vi "Multi-Point Tracking.vi"() -> ()   [LabVIEW 2021]
uses:
  <vilib>/myRIO/Instrument Drivers/Onboard IO/I2C/typedefs/I2C User Configuration.ctl
  <vilib>/myRIO/Instrument Drivers/Onboard IO/I2C/typedefs/I2C Transfer Rate.ctl
  <vilib>/myRIO/Instrument Drivers/Onboard IO/I2C/typedefs/I2C Reference.ctl
  <vilib>/myRIO/Common/Instrument Driver Framework/Utilities/typedefs/myRIO Generic Hardware Reference.ctl
  <vilib>/myRIO/Common/Instrument Driver Framework/Utilities/typedefs/Hardware Version Enum.ctl
  <vilib>/myRIO/Common/Instrument Driver Framework/Utilities/typedefs/myRIO v1.0 Reference.ctl
  <vilib>/myRIO/Common/Instrument Driver Framework/Utilities/typedefs/Generic FPGA Reference.ctl
  <vilib>/myRIO/Common/Instrument Driver Framework/myRIO v1.0/I2C/typedefs/I2C Channels Enum.ctl
  <vilib>/myRIO/Instrument Drivers/Onboard IO/I2C/typedefs/I2C Configuration.ctl
  <vilib>/userDefined/High Color/nirio_resource_hc.ctl
  <vilib>/myRIO/Instrument Drivers/Onboard IO/PWM/typedefs/PWM Reference.ctl
  <vilib>/myRIO/Common/Instrument Driver Framework/myRIO v1.0/PWM/typedefs/PWM Channels Enum.ctl
  <vilib>/myRIO/Instrument Drivers/Onboard IO/PWM/typedefs/PWM Configuration.ctl
  <vilib>/myRIO/Common/Instrument Driver Framework/myRIO v1.0/Encoder/typedefs/Encoder Signal Mode.ctl
  <vilib>/myRIO/Instrument Drivers/Onboard IO/Encoder/typedefs/Encoder Reference.ctl
  <vilib>/myRIO/Common/Instrument Driver Framework/myRIO v1.0/Encoder/typedefs/Encoder Channels Enum.ctl
  <vilib>/myRIO/Common/Instrument Driver Framework/myRIO v1.0/Encoder/typedefs/Encoder Configuration v1.0.ctl
  <vilib>/myRIO/Instrument Drivers/Onboard IO/DIO/typedefs/DIO Reference.ctl
  <vilib>/myRIO/Common/Instrument Driver Framework/myRIO v1.0/DIO/typedefs/DIO Channels List.ctl
  <vilib>/myRIO/Common/Instrument Driver Framework/myRIO v1.0/DIO/typedefs/DIO Channels Enum.ctl
  <vilib>/myRIO/Common/Instrument Driver Framework/Utilities/vis/Is FPGA Ref Available.vi
  <vilib>/myRIO/Common/Instrument Driver Framework/myRIO v1.0/I2C/vis/myRIO v1.1 Open I2C.vi
  <vilib>/myRIO/Instrument Drivers/Onboard IO/I2C/vis/Configure.vi
  <vilib>/myRIO/Instrument Drivers/Onboard IO/I2C/vis/Write.vi
  <vilib>/myRIO/Common/Instrument Driver Framework/myRIO v1.0/Encoder/vis/myRIO v1.1 Open Encoder.vi
  <vilib>/myRIO/Instrument Drivers/Onboard IO/Encoder/vis/Read.vi
  <vilib>/myRIO/Common/Instrument Driver Framework/myRIO v1.0/PWM/vis/myRIO v1.1 Open PWM.vi
  <vilib>/myRIO/Instrument Drivers/Onboard IO/PWM/vis/Set Duty Cycle and Frequency.vi
  <vilib>/myRIO/Common/Instrument Driver Framework/myRIO v1.0/DIO/vis/myRIO v1.1 Open DIO.vi
  <vilib>/myRIO/Instrument Drivers/Onboard IO/DIO/vis/Write.vi
  <vilib>/myRIO/Instrument Drivers/Onboard IO/I2C/vis/Write Read.vi
  <vilib>/Analysis/baseanly.llb/Mean (DBL).vi
  <vilib>/myRIO/Common/Instrument Driver Framework/Utilities/vis/Validate Channels.vi
  <vilib>/myRIO/Common/Instrument Driver Framework/myRIO v1.0/I2C/vis/myRIO v1.0 Reserve I2C.vi
  <vilib>/myRIO/Common/Instrument Driver Framework/myRIO v1.0/Encoder/vis/myRIO v1.0 Reserve Encoder.vi
  <vilib>/myRIO/Common/Instrument Driver Framework/myRIO v1.0/PWM/vis/myRIO v1.0 Reserve PWM.vi
  <vilib>/myRIO/Common/Instrument Driver Framework/myRIO v1.0/DIO/vis/myRIO v1.0 Reserve DIO.vi
  <vilib>/myRIO/Common/Instrument Driver Framework/myRIO v1.0/UART/vis/myRIO v1.0 Close UART.vi
  <vilib>/myRIO/Common/Instrument Driver Framework/myRIO v1.0/I2C/vis/myRIO v1.0 Build MUX Configuration I2C.vi
  <vilib>/myRIO/Common/Instrument Driver Framework/myRIO v1.0/Resource Manager/vis/myRIO v1.0 Reserve Channel List.vi
  <vilib>/myRIO/Common/Instrument Driver Framework/myRIO v1.0/Encoder/vis/myRIO v1.0 Build MUX Configuration Encoder.vi
  <vilib>/myRIO/Common/Instrument Driver Framework/myRIO v1.0/PWM/vis/myRIO v1.0 Build MUX Configuration PWM.vi
  <vilib>/myRIO/Common/Instrument Driver Framework/myRIO v1.0/DIO/vis/myRIO v1.0 Build MUX Configuration DIO.vi
  <vilib>/myRIO/Common/Instrument Driver Framework/myRIO v1.0/Resource Manager/vis/myRIO v1.0 Create Configuration List.vi
  <vilib>/myRIO/Common/Instrument Driver Framework/myRIO v1.0/Resource Manager/vis/myRIO v1.0 Reserve Channel.vi
  <vilib>/myRIO/Common/Instrument Driver Framework/myRIO v1.0/Resource Manager/vis/myRIO v1.0 Unreserve Channel.vi
  <vilib>/myRIO/Common/Instrument Driver Framework/myRIO v1.0/Resource Manager/vis/myRIO v1.0 Build Mutex Name.vi
  <vilib>/Utility/VariantDataType/GetNumericInfo.vi
  <vilib>/Utility/error.llb/Error Cluster From Error Code.vi
  <vilib>/myRIO/Common/Instrument Driver Framework/myRIO v1.0/myRIO v1.1 Open.vi
  <vilib>/myRIO/Common/Instrument Driver Framework/Utilities/vis/IO Manager.vi
  <vilib>/myRIO/Common/Instrument Driver Framework/Utilities/vis/Configuration Manager.vi
  <vilib>/myRIO/Common/Instrument Driver Framework/myRIO v1.0/Resource Manager/vis/myRIO v1.0 Configure IO.vi
  <vilib>/myRIO/Common/Instrument Driver Framework/myRIO v1.0/myRIO v1.0 Close.vi
  <vilib>/myRIO/Common/Instrument Driver Framework/myRIO v1.0/I2C/vis/myRIO v1.0 Configure I2C.vi
  <vilib>/myRIO/Common/Instrument Driver Framework/myRIO v1.0/I2C/vis/myRIO v1.0 Write I2C.vi
  <vilib>/myRIO/Common/Instrument Driver Framework/myRIO v1.0/Encoder/vis/myRIO v1.0 Configure Encoder.vi
  <vilib>/myRIO/Common/Instrument Driver Framework/myRIO v1.0/Encoder/vis/myRIO v1.0 Read Encoder.vi
  <vilib>/addons/Fuzzy Logic/FL Fuzzy Controller (SISO).vi
  <vilib>/myRIO/Common/Instrument Driver Framework/myRIO v1.0/PWM/vis/myRIO v1.0 Write PWM.vi
  <vilib>/myRIO/Common/Instrument Driver Framework/myRIO v1.0/DIO/vis/myRIO v1.0 Write DIO.vi
  <vilib>/myRIO/Common/Instrument Driver Framework/myRIO v1.0/I2C/vis/myRIO v1.0 Read I2C.vi
  <vilib>/myRIO/Common/Instrument Driver Framework/Utilities/vis/FPGA Ref Manager.vi
  <vilib>/myRIO/Common/Instrument Driver Framework/myRIO v1.0/myRIO v1.0 Reset FPGA.vi
  <vilib>/myRIO/Common/Instrument Driver Framework/myRIO v1.0/IRQ/vis/myRIO v1.0 IRQ Info FGV.vi
  <vilib>/myRIO/Common/Instrument Driver Framework/myRIO v1.0/IRQ/vis/myRIO v1.0 Timer IRQ Info FGV.vi
  <vilib>/myRIO/Common/Instrument Driver Framework/myRIO v1.0/IRQ/vis/myRIO v1.0 ISR Agent.vi
  <vilib>/myRIO/Instrument Drivers/Utilities/vis/Reset Index.vi
  <vilib>/myRIO/Common/Instrument Driver Framework/myRIO v1.0/Resource Manager/vis/myRIO v1.0 Block Write Resource Manager.vi
  <vilib>/myRIO/Express VI/Onboard IO/I2C/I2C Express VI.xnode
  <vilib>/myRIO/Instrument Drivers/Onboard IO/I2C/vis/myRIO I2C Open.xnode
  <vilib>/myRIO/Express VI/Onboard IO/Encoder/Encoder Express VI.xnode
  <vilib>/myRIO/Instrument Drivers/Onboard IO/Encoder/vis/myRIO Encoder Open.xnode
  <vilib>/myRIO/Common/Instrument Driver Framework/myRIO v1.0/Encoder/typedefs/Encoder Count Direction Enum.ctl
  <vilib>/myRIO/Express VI/Onboard IO/PWM/PWM Express VI.xnode
  <vilib>/myRIO/Instrument Drivers/Onboard IO/PWM/vis/myRIO PWM Open.xnode
  <vilib>/myRIO/Express VI/Onboard IO/DO/DO Express VI.xnode
  <vilib>/myRIO/Instrument Drivers/Onboard IO/DIO/vis/myRIO DIO Open.xnode
  <vilib>/myRIO/Instrument Drivers/Onboard IO/I2C/I2C.lvlib
  <vilib>/ptbypt/NI_PtbyPt.lvlib
  <vilib>/myRIO/Instrument Drivers/Onboard IO/PWM/PWM.lvlib
  <vilib>/myRIO/Instrument Drivers/Onboard IO/DIO/DIO.lvlib
  <vilib>/myRIO/Instrument Drivers/Utilities/Utilities.lvlib
  <vilib>/myRIO/Instrument Drivers/Onboard IO/Encoder/Encoder.lvlib
  <vilib>/Analysis/NI_AALBase.lvlib
  <vilib>/addons/Fuzzy Logic/NI_Fuzzy_Logic_API.lvlib
panel:
  out "correct gz":dbl
  out "correct GZ":dbl format="%0.2f"
  out "速度":dbl
  out "單位距離":dbl
  out "總行程":dbl
  out "右圈數":dbl
  out "左圈數":dbl
  out "Reset counter":bool
  out "Velocity(cm/sec)":cluster{dbl[], dbl[]}(graph)
  in  "array":dbl[][](array[numeric])
  out "output cluster":cluster{"Array 2":dbl[], "Array 2":dbl[]}
  out "appended array":dbl[][](array[numeric])
  out "path5":cluster{dbl[], dbl[]}(graph)
  out "distance":dbl
  out "Yaw target":dbl
  out "Yt":dbl
  out "Xt":dbl
  out "Yg":dbl
  out "Xg":dbl
  out "P-gain":dbl
  out "Error":cluster{dbl[], dbl[]}(graph)
  out "Yaw error":dbl
  out "Command/Gauge":cluster{dbl[], dbl[]}[](graph)
  out "angular degree":dbl format="%0.2f"
  out "Velocity duty cycle":dbl(slide) scale=0.0..1.0
  out "Turn duty cycle":dbl(slide) scale=0.0..1.0
  in  "start":bool
  in  "remote":bool
  out "Guage":dbl(knob) scale=0.0..360.0
  out "GZ":dbl format="%0.2f"
  in  "G 歸零":bool
  in  "G 校正":bool
  in  "stop":bool
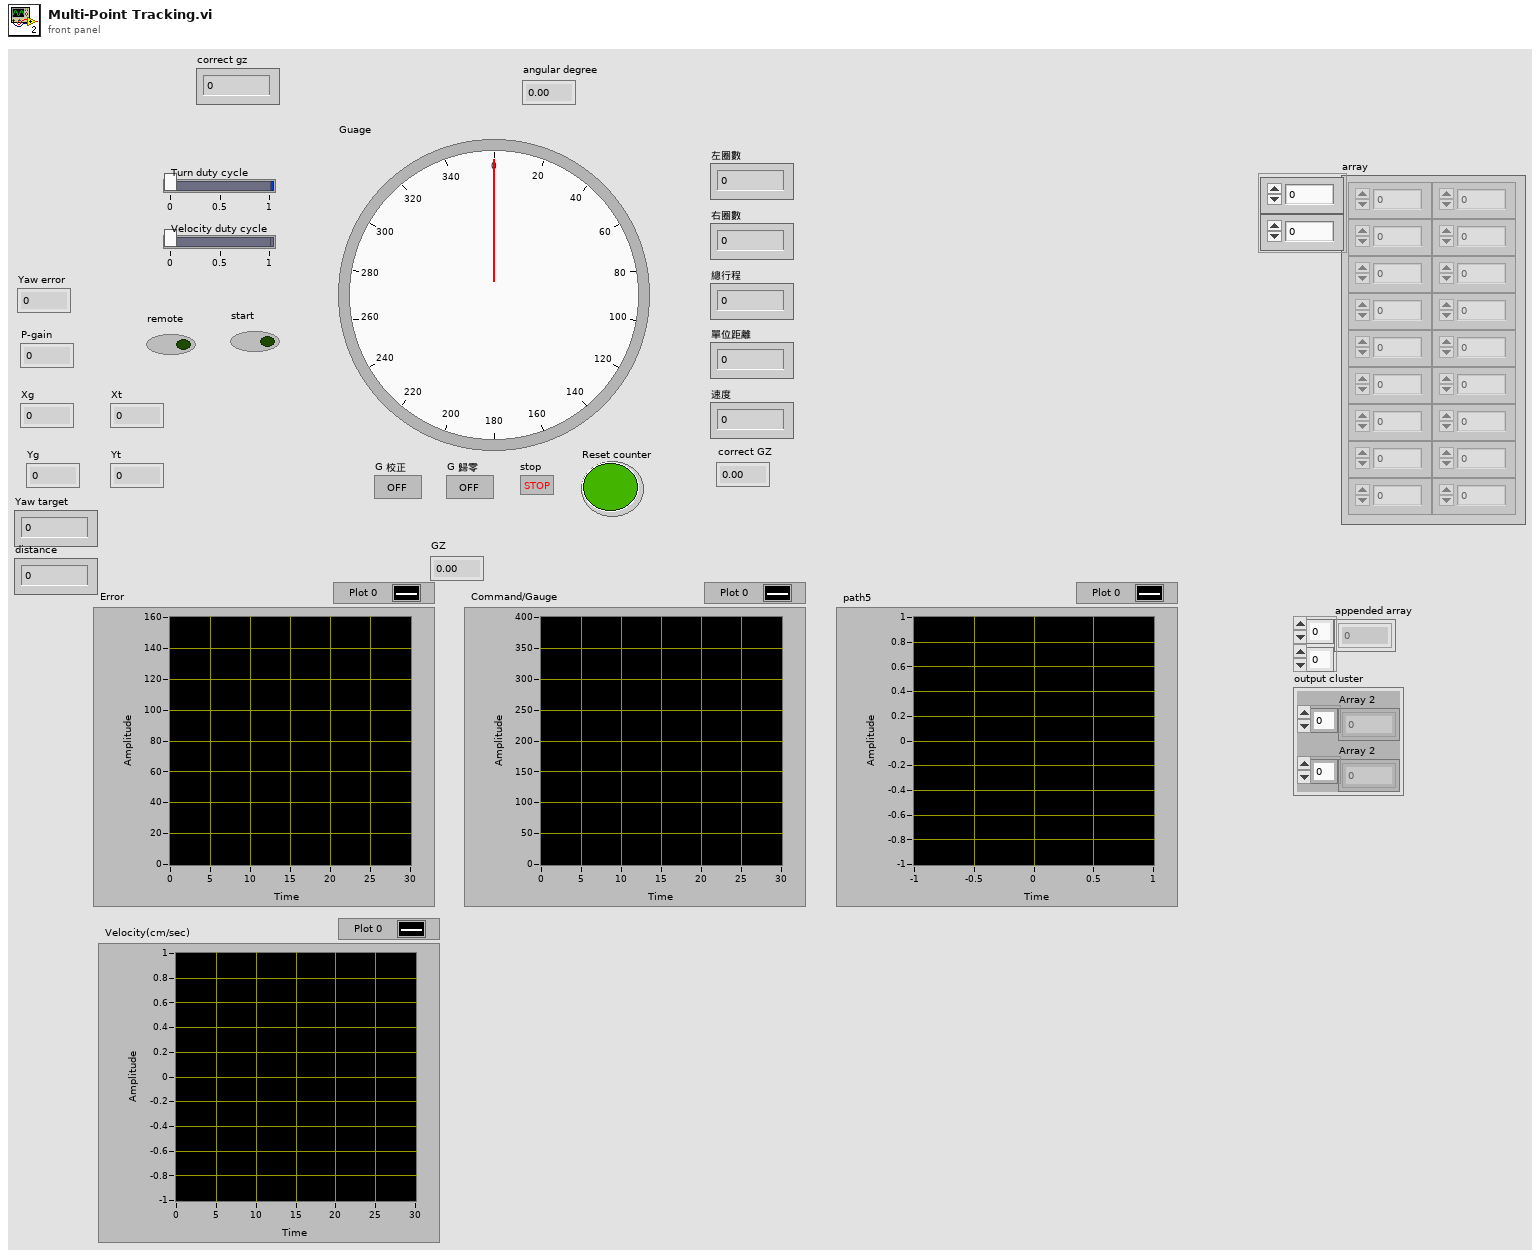
[diagram p1: front panel]
types:
  T1 = typedef "I2C.lvlib/I2C Reference.ctl" = cluster{"myRIO Reference":T2, "I2C Channels Enum":T6, "I2C Configuration":T7}
  T2 = typedef "myRIO Generic Hardware Reference.ctl" = cluster{"myRIO Model":T3, "myRIO Hardware Reference":T4}
  T3 = typedef "Hardware Version Enum.ctl" = enum16{"Unknown", "myRIO-1900", "myRIO-1950", "roboRIO", "NI ELVIS RIO CM", "ELVIS III"}
  T4 = typedef "myRIO v1.0 Reference.ctl" = cluster{"Generic FPGA Reference":T5, "Allow multiple opens":bool}
  T5 = typedef "Generic FPGA Reference.ctl" = refnum<k20>
  T6 = typedef "I2C Channels Enum.ctl" = enum16{"Not Connected", "A/I2C", "B/I2C", "I2C/I2C"}
  T7 = typedef "I2C.lvlib/I2C Configuration.ctl" = cluster{"I2C Transfer Rate":T8}
  T8 = typedef "I2C.lvlib/I2C Transfer Rate.ctl" = enum16{"Standard mode (100 kbps)", "Fast mode (400 kbps)"}
  T9 = typedef "I2C.lvlib/I2C User Configuration.ctl" = cluster{"I2C Transfer Rate":T8}
  T10 = typedef "nirio_resource_hc.ctl" = tag
  T11 = typedef "Encoder.lvlib/Encoder Reference.ctl" = cluster{"myRIO Reference":T2, "Encoder Channels Enum":T12}
  T12 = typedef "Encoder Channels Enum.ctl" = enum16{"Not Connected", "C/ENC0", "C/ENC1", "A/ENC", "A/ENC0", "A/ENC1", "A/ENC2", "A/ENC3", "A/ENC4", "A/ENC5", "A/ENC6", "A/ENC7", "A/ENC8", "A/ENC9", "B/ENC", "B/ENC0", "B/ENC1", "B/ENC2", "B/ENC3", "B/ENC4", "B/ENC5", "B/ENC6", "B/ENC7", "B/ENC8", "B/ENC9", "DIO/ENC0", "DIO/ENC1", "DIO/ENC2", "DIO/ENC3", "DIO/ENC4"}
  T13 = typedef "Encoder Signal Mode.ctl" = enum16{"Quadrature phase signal", "Step and direction signal"}
  T14 = typedef "DIO.lvlib/DIO Reference.ctl" = cluster{"myRIO Reference":T2, "DIO Channels List":T15}
  T15 = typedef "DIO Channels List.ctl" = T16[]
  T16 = typedef "DIO Channels Enum.ctl" = enum16{"Not Connected", "C/DIO0", "C/DIO1", "C/DIO2", "C/DIO3", "C/DIO4", "C/DIO5", "C/DIO6", "C/DIO7", "A/DIO0", "A/DIO1", "A/DIO2", "A/DIO3", "A/DIO4", "A/DIO5", "A/DIO6", "A/DIO7", "A/DIO8", "A/DIO9", "A/DIO10", "A/DIO11", "A/DIO12", "A/DIO13", "A/DIO14", "A/DIO15", "A/DIO16", "A/DIO17", "A/DIO18", "A/DIO19", "B/DIO0", "B/DIO1", "B/DIO2", "B/DIO3", "B/DIO4", "B/DIO5", "B/DIO6", "B/DIO7", "B/DIO8", "B/DIO9", "B/DIO10", "B/DIO11", "B/DIO12", "B/DIO13", "B/DIO14", "B/DIO15", "B/DIO16", "B/DIO17", "B/DIO18", "B/DIO19", "LED0", "LED1", "LED2", "LED3", "Button0", "DIO/DIO0", "DIO/DIO1", "DIO/DIO2", "DIO/DIO3", "DIO/DIO4", "DIO/DIO5", "DIO/DIO6", "DIO/DIO7", "DIO/DIO8", "DIO/DIO9", "SPI/CS0", "SPI/CS1", "SPI/CS2", "SPI/CS3", "LED RADIO (Green)", "LED RADIO (Red)", "LED COMM (Green)", "LED COMM (Red)", "LED MODE (Green)", "LED MODE (Red)"}
  T17 = typedef "PWM.lvlib/PWM Reference.ctl" = cluster{"myRIO Reference":T2, "PWM Channels Enum":T18, "PWM Configuration":T19}
  T18 = typedef "PWM Channels Enum.ctl" = enum16{"Not Connected", "C/PWM0", "C/PWM1", "A/PWM0", "A/PWM1", "A/PWM2", "A/PWM3", "A/PWM4", "A/PWM5", "A/PWM6", "A/PWM7", "A/PWM8", "A/PWM9", "A/PWM10", "A/PWM11", "A/PWM12", "A/PWM13", "A/PWM14", "A/PWM15", "A/PWM16", "A/PWM17", "A/PWM18", "A/PWM19", "B/PWM0", "B/PWM1", "B/PWM2", "B/PWM3", "B/PWM4", "B/PWM5", "B/PWM6", "B/PWM7", "B/PWM8", "B/PWM9", "B/PWM10", "B/PWM11", "B/PWM12", "B/PWM13", "B/PWM14", "B/PWM15", "B/PWM16", "B/PWM17", "B/PWM18", "B/PWM19", "PWM/PWM0", "PWM/PWM1", "PWM/PWM2", "PWM/PWM3", "PWM/PWM4", "PWM/PWM5", "PWM/PWM6", "PWM/PWM7", "PWM/PWM8", "PWM/PWM9"}
  T19 = typedef "PWM.lvlib/PWM Configuration.ctl" = cluster{"Frequency":dbl, "Duty Cycle":dbl}
  T20 = typedef "NI_Fuzzy_Logic_API.lvlib/FL System.ctl" = cluster{"input variables":T21[], "output variables":T21[], "rules":T24[], "defuzzification method":T30, "description":string, "user MF interpolating polynomials":T31[]}
  T21 = typedef "NI_Fuzzy_Logic_API.lvlib/FL Variable.ctl" = cluster{"name":string, "range":dbl[], "MFs":T22[]}
  T22 = typedef "NI_Fuzzy_Logic_API.lvlib/FL Membership Function.ctl" = cluster{"name":string, "shape":T23, "points":dbl[], "color":u32, "user-defined shape index":i32}
  T23 = typedef "NI_Fuzzy_Logic_API.lvlib/FL Membership Function Shape.ctl" = u16
  T24 = typedef "NI_Fuzzy_Logic_API.lvlib/FL Rule.ctl" = cluster{"antecedents":T25[], "antecedent connective":T27, "consequents":T28[], "consequent implication":T29, "degree of support":dbl}
  T25 = typedef "NI_Fuzzy_Logic_API.lvlib/FL Antecedent.ctl" = cluster{"Var Index":i32, "MF Index":i32, "Cond":T26}
  T26 = typedef "NI_Fuzzy_Logic_API.lvlib/FL Modifier.ctl" = u16
  T27 = typedef "NI_Fuzzy_Logic_API.lvlib/FL Antecedent Connective.ctl" = u16
  T28 = typedef "NI_Fuzzy_Logic_API.lvlib/FL Consequent.ctl" = cluster{"Var Index":i32, "MF Index":i32, "Cond":T26}
  T29 = typedef "NI_Fuzzy_Logic_API.lvlib/FL Consequent Implication.ctl" = u16
  T30 = typedef "NI_Fuzzy_Logic_API.lvlib/FL Defuzzification.ctl" = u16
  T31 = typedef "NI_Fuzzy_Logic_API.lvlib/FL Interpolating polynomials.ctl" = cluster{"X":dbl[], "Y":dbl[], "Y(x) coeff":dbl[][], "X(y) coeff":dbl[][], "Area(y) coeff":dbl[][], "coa_x(y) coeff":dbl[][]}
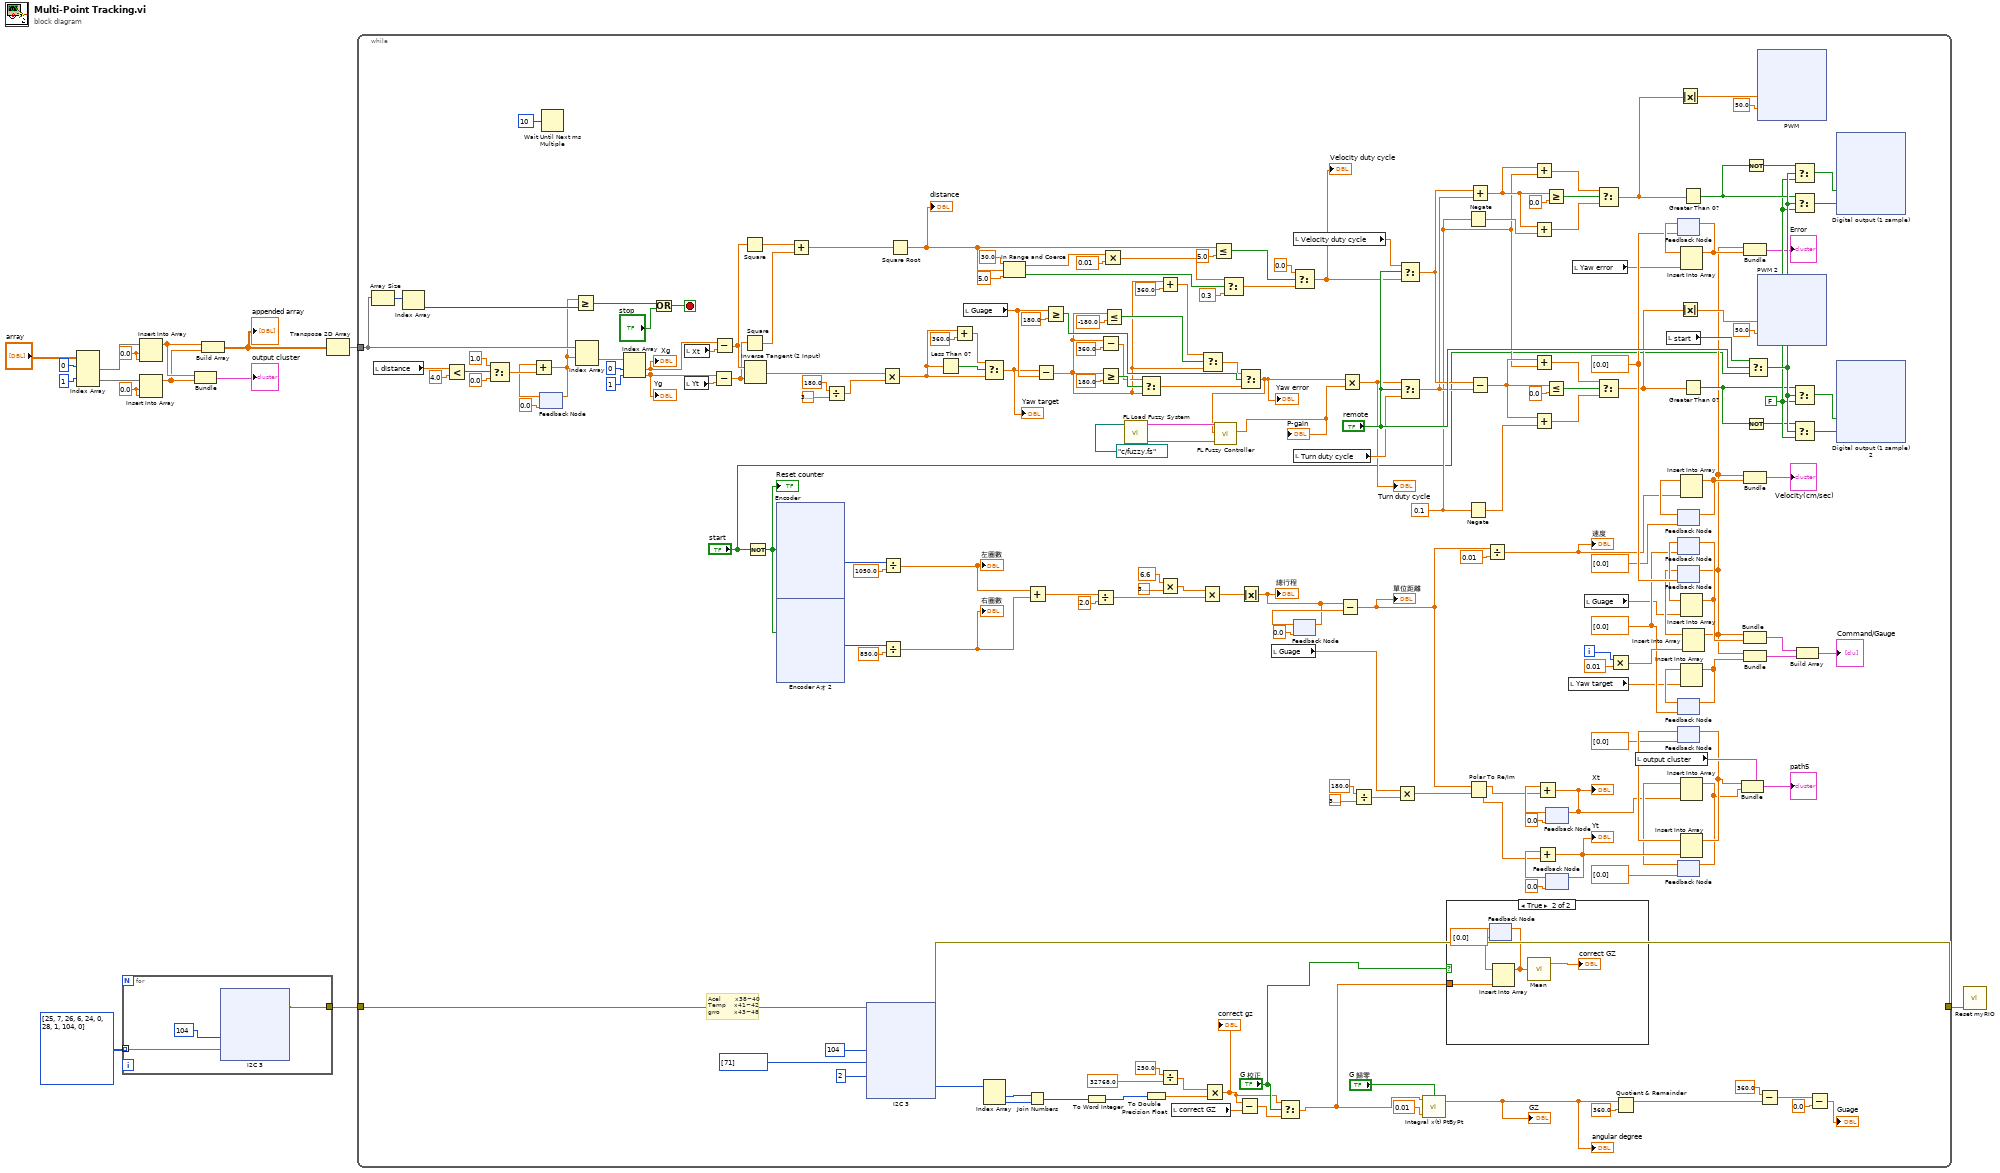
[diagram p0: block diagram]
diagram:
  w1 = 0.0 ("new element/subarray")
  w3 = 0.0 ("new element/subarray")
  n1 = Index Array(array="array", index (row) #1=0 ("index (row)"), index (row) #2=1 ("index (row)")) -> (element #1=w7:dbl[], element #2=w6:dbl[])  [unwired: 2 in]
  n2 = for {
    tunnel: u8[][] [[25, 7], [26, 6], [24, 0], [28, 1], [104, 0]] ("Bytes to Write") -> [w16] mode=indexing
    tunnel: [w18] -> w14
    n3 = xnode "I2C 3"("Slave Address (7-bit)"=u8 104, "Bytes to Write"=w16) -> ("error out"=w18:errorcluster)  [unwired: 1 in]
  }
  n4 = Insert Into Array(array=w7, index=w3, new element=w3) -> (w4:dbl[])
  n5 = Insert Into Array(array=w6, index=w1, new element=w1) -> (w2:dbl[])
  n6 = Bundle("array"=w4, "array"=w2) -> (→"output cluster":cluster{"array":dbl[], "array":dbl[]})  [unwired: 1 in]
  n7 = Build Array(w4, w2) -> (w12:dbl[][])
  "appended array" <- w12
  n8 = Transpose 2D Array(2D array=w12) -> (transposed array=w10:dbl[][])
  n9 = while {
    tunnel: w14 -> [w77]
    tunnel: [w76] -> w13
    tunnel: w10 -> [w117]
    i -> [w218]
    stop <- w242 stop-if-true
    w185 = 0.1 ("y")
    w220 = dbl[] [0.0]
    w225 = dbl[] [0.0]
    w232 = FALSE
    # "Acel       x38~40\nTemp    x41~42\ngrro       x43~48"
    n10 = Array Size(array=w117) -> (size(s)=w116:i32[])
    n11 = local read "distance"() -> (w127:dbl)
    n12 = Index Array(array=w116) -> (element=w115:i32)  [unwired: 1 in]
    n13 = Less?(x=w127, y=4.0) -> (x < y?=w125:bool)
    n14 = Select(t=1.0, s=w125, f=0.0) -> (s? t:f=w122:dbl)
    n15 = feedback #1(0.0) -> (w121:dbl)
    n16 = Add(x=w121, y=w122) -> (x+y=w114:dbl)
    n17 = feedback-in #1(w114) -> ()
    n18 = Wait Until Next ms Multiple(millisecond multiple=u32 10) -> ()  [unwired: 1 out]
    n19 = Greater Or Equal?(x=w114, y=w115) -> (x >= y?=w119:bool)
    n20 = Index Array(array=w117, index (row)=w114) -> (element=w118:dbl[])  [unwired: 1 in]
    n21 = Index Array(array=w118, index #1=0 ("index"), index #2=1 ("index")) -> (element #1=w111:dbl, element #2=w110:dbl)
    "Yg" <- w110
    "Xg" <- w111
    n22 = Or(x=w119, y="stop") -> (x .or. y?=w242:bool)
    n23 = local read "Xt"() -> (w171:dbl)
    n24 = local read "Yt"() -> (w170:dbl)
    n25 = Subtract(x=w110, y=w170) -> (x-y=w168:dbl)
    n26 = Subtract(x=w111, y=w171) -> (x-y=w169:dbl)
    n27 = Square(x=w169) -> (x^2=w167:dbl)
    n28 = Square(x=w168) -> (x^2=w166:dbl)
    n29 = Inverse Tangent (2 Input)(1:w168, 2:w169) -> (0:w164:dbl)
    n30 = Not(x="start") -> (.not. x?=w101:bool)
    "Reset counter" <- w101
    n31 = xnode "Encoder"("Reset Counter"=w101) -> ("Counter Value"=w97:i32)  [unwired: 1 in, 3 out]
    n32 = xnode "Encoder Aオ 2"("Reset Counter"=w101) -> ("Counter Value"=w98:i32)  [unwired: 1 in, 3 out]
    n33 = Add(x=w167, y=w166) -> (x+y=w165:dbl)
    n34 = Divide(x=180.0, y=3.141592653589793) -> (x/y=w161:dbl)
    n35 = xnode "I2C 3"("Slave Address (7-bit)"=u8 104, "Bytes to Write"=u8[] [71], "Byte Count"=u32 2, "error in (no error)"=w77) -> ("Bytes Read"=w72:u8[], "error out"=w76:errorcluster)
    n36 = Multiply(x=w164, y=w161) -> (x*y=w159:dbl)
    n37 = Divide(x=w97, y=1050.0) -> (x/y=w96:dbl)
    "左圈數" <- w96
    n38 = Divide(x=w98, y=850.0) -> (x/y=w95:dbl)
    "右圈數" <- w95
    n39 = Square Root(x=w165) -> (sqrt(x)=w148:dbl)
    "distance" <- w148
    n40 = Less Than 0?(x=w159) -> (x < 0?=w160:bool)
    n41 = Add(x=w159, y=360.0) -> (x+y=w157:dbl)
    n42 = local read "Guage"() -> (w172:dbl)
    n43 = Select(t=w157, s=w160, f=w159) -> (s? t:f=w156:dbl)
    "Yaw target" <- w156
    n44 = Index Array(array=w72) -> (element #1=w255:u8, element #2=w254:u8)  [unwired: 2 in]
    n45 = In Range and Coerce(upper limit=30.0, x=w148, lower limit=5.0) -> (coerced(x)=w153:dbl, In Range?=w151:bool)
    n46 = Add(x=w96, y=w95) -> (x+y=w94:dbl)
    n47 = Join Numbers(hi=w255, lo=w254) -> ((hi.lo)=w253:u16)
    n48 = Subtract(x=w156, y=w172) -> (x-y=w199:dbl)
    n49 = Greater Or Equal?(x=w172, y=180.0) -> (x >= y?=w205:bool)
    n50 = To Word Integer(number=w253) -> (16bit integer=w250:i16)
    n51 = Divide(x=w94, y=2.0) -> (x/y=w89:dbl)
    n52 = Subtract(x=w199, y=360.0) -> (x-y=w200:dbl)
    n53 = Greater Or Equal?(x=w199, y=180.0) -> (x >= y?=w207:bool)
    n54 = Multiply(x=w153, y=0.01) -> (x*y=w150:dbl)
    n55 = Less Or Equal?(x=w199, y=-180.0) -> (x <= y?=w208:bool)
    n56 = call <vilib>:"FL Load Fuzzy System.vi"("file path"=path "c:/fuzzy.fs") -> ("error out"=w64:errorcluster, "fuzzy system out"=w65:T20)  [unwired: 9 in]
    n57 = Select(t=w200, s=w207, f=w199) -> (s? t:f=w201:dbl)
    n58 = To Double Precision Float(number=w250) -> (double precision float=w243:dbl)
    n59 = Add(x=w199, y=360.0) -> (x+y=w198:dbl)
    n60 = Multiply(x=6.6, y=3.141592653589793) -> (x*y=w90:dbl)
    n61 = Divide(x=250.0, y=32768.0) -> (x/y=w249:dbl)
    n62 = local read "correct GZ"() -> (w70:dbl)
    n63 = Multiply(x=w90, y=w89) -> (x*y=w88:dbl)
    n64 = Select(t=w198, s=w208, f=w199) -> (s? t:f=w202:dbl)
    n65 = Multiply(x=w249, y=w243) -> (x*y=w68:dbl)
    "correct gz" <- w68
    n66 = Less Or Equal?(x=w148, y=5.0) -> (x <= y?=w146:bool)
    n67 = Select(t=w150, s=w151, f=0.3) -> (s? t:f=w145:dbl)
    n68 = Subtract(x=w68, y=w70) -> (x-y=w67:dbl)
    n69 = Select(t=w202, s=w205, f=w201) -> (s? t:f=w63:dbl)
    "Yaw error" <- w63
    n70 = call-poly <vilib>:"FL Fuzzy Controller.vi"("error in (no error)"=w64, "input value"=w63, "fuzzy system in"=w65) -> ("output value"=w62:dbl)  [unwired: 4 in, 4 out]
    "P-gain" <- w62
    n71 = Absolute Value(x=w88) -> (abs(x)=w85:dbl)
    "總行程" <- w85
    n72 = local read "Guage"() -> (w142:dbl)
    n73 = Select(t=w68, s="G 校正", f=w67) -> (s? t:f=w66:dbl)
    n74 = local read "Velocity duty cycle"() -> (w178:dbl)
    n75 = Select(t=0.0, s=w146, f=w145) -> (s? t:f=w143:dbl)
    "Velocity duty cycle" <- w143
    n76 = local read "Turn duty cycle"() -> (w197:dbl)
    n77 = feedback-in #2(w85) -> ()
    n78 = feedback #2(0.0) -> (w86:dbl)
    n79 = Subtract(x=w85, y=w86) -> (x-y=w84:dbl)
    "單位距離" <- w84
    n80 = Multiply(x=w63, y=w62) -> (x*y=w177:dbl)
    "Turn duty cycle" <- w177
    n81 = Divide(x=180.0, y=3.141592653589793) -> (x/y=w139:dbl)
    n82 = Multiply(x=w142, y=w139) -> (x*y=w138:dbl)
    n83 = Select(t=w178, s="remote", f=w143) -> (s? t:f=w196:dbl)
    n84 = Select(t=w177, s="remote", f=w197) -> (s? t:f=w195:dbl)
    n85 = call <vilib>:"Integral x(t) PtByPt.vi"("initialize"="G 歸零", "dt"=0.01, "x"=w66) -> ("integral x(t)"=w247:dbl)  [unwired: 1 in, 1 out]
    "GZ" <- w247
    "angular degree" <- w247
    n86 = case shown="True" "G 校正" {
      tunnel: w66 -> [_ w256]
      frame False {
      }
      frame True {
        n87 = feedback #3(dbl[] [0.0]) -> (w260:dbl[])
        n88 = Insert Into Array(array=w260, new element=w256) -> (w259:dbl[])  [unwired: 1 in]
        n89 = feedback-in #3(w259) -> ()
        n90 = call-poly <vilib>:"Mean.vi"("X"=w259) -> ("mean"=→"correct GZ":dbl)  [unwired: 1 out]
      }
    }
    n91 = Negate(x=w185) -> (-x=w190:dbl)
    n92 = Negate(x=w185) -> (-x=w184:dbl)
    n93 = Polar To Re/Im(2:w138, 3:w84) -> (0:w59:dbl, 1:w60:dbl)
    n94 = Add(x=w196, y=w195) -> (x+y=w191:dbl)
    n95 = Subtract(x=w196, y=w195) -> (x-y=w187:dbl)
    n96 = Divide(x=w84, y=0.01) -> (x/y=w82:dbl)
    "速度" <- w82
    n97 = Add(x=w191, y=w185) -> (x+y=w188:dbl)
    n98 = Add(x=w191, y=w190) -> (x+y=w189:dbl)
    n99 = Add(x=w187, y=w185) -> (x+y=w186:dbl)
    n100 = Add(x=w187, y=w184) -> (x+y=w183:dbl)
    n101 = Greater Or Equal?(x=w191, y=0.0) -> (x >= y?=w192:bool)
    n102 = Less Or Equal?(x=w187, y=0.0) -> (x <= y?=w182:bool)
    n103 = feedback #4(0.0) -> (w132:dbl)
    n104 = Add(x=w132, y=w60) -> (x+y=w128:dbl)
    "Xt" <- w128
    n105 = feedback-in #4(w128) -> ()
    n106 = feedback #5(0.0) -> (w137:dbl)
    n107 = Add(x=w137, y=w59) -> (x+y=w135:dbl)
    "Yt" <- w135
    n108 = feedback-in #5(w135) -> ()
    n109 = local read "Yaw target"() -> (w212:dbl)
    n110 = local read "Yaw error"() -> (w211:dbl)
    n111 = local read "Guage"() -> (w173:dbl)
    n112 = Select(t=w188, s=w192, f=w189) -> (s? t:f=w180:dbl)
    n113 = Select(t=w186, s=w182, f=w183) -> (s? t:f=w181:dbl)
    n114 = Multiply(x=w218, y=0.01) -> (x*y=w227:dbl)
    n115 = Quotient & Remainder(x=w247, y=360.0) -> (x-y*floor(x/y)=w245:dbl)  [unwired: 1 out]
    n116 = local read "output cluster"() -> (w108:cluster{"Array 2":dbl[], "Array 2":dbl[]})
    n117 = local read "start"() -> (w179:bool)
    n118 = feedback #6(w225) -> (w226:dbl[])
    n119 = feedback #7(dbl[] [0.0]) -> (w107:dbl[])
    n120 = feedback #8(w220) -> (w222:dbl[])
    n121 = feedback #9(w225) -> (w219:dbl[])
    n122 = feedback #10(w220) -> (w221:dbl[])
    n123 = feedback #11(dbl[] [0.0]) -> (w134:dbl[])
    n124 = feedback #12(dbl[] [0.0]) -> (w130:dbl[])
    n125 = Absolute Value(x=w180) -> (abs(x)=w240:dbl)
    n126 = Absolute Value(x=w181) -> (abs(x)=w239:dbl)
    n127 = Insert Into Array(array=w226, new element=w211) -> (w224:dbl[])  [unwired: 1 in]
    n128 = feedback-in #6(w224) -> ()
    n129 = Insert Into Array(array=w107, new element=w82) -> (w105:dbl[])  [unwired: 1 in]
    n130 = feedback-in #7(w105) -> ()
    n131 = Insert Into Array(array=w222, new element=w173) -> (w217:dbl[])  [unwired: 1 in]
    n132 = feedback-in #8(w217) -> ()
    n133 = Insert Into Array(array=w221, new element=w212) -> (w216:dbl[])  [unwired: 1 in]
    n134 = feedback-in #10(w216) -> ()
    n135 = Insert Into Array(array=w130, new element=w128) -> (w57:dbl[])  [unwired: 1 in]
    n136 = feedback-in #12(w57) -> ()
    n137 = Insert Into Array(array=w134, new element=w135) -> (w58:dbl[])  [unwired: 1 in]
    n138 = feedback-in #11(w58) -> ()
    n139 = Greater Than 0?(x=w180) -> (x > 0?=w233:bool)
    n140 = Greater Than 0?(x=w181) -> (x > 0?=w230:bool)
    n141 = Insert Into Array(array=w219, new element=w227) -> (w104:dbl[])  [unwired: 1 in]
    n142 = feedback-in #9(w104) -> ()
    n143 = Bundle(cluster=w108, "Array 2"=w58, "Array 2"=w57) -> (→"path5":cluster{"Array 2":dbl[], "Array 2":dbl[]})
    n144 = Bundle(w104, w224) -> (→"Error":cluster{dbl[], dbl[]})  [unwired: 1 in]
    n145 = Bundle(w104, w105) -> (→"Velocity(cm/sec)":cluster{dbl[], dbl[]})  [unwired: 1 in]
    n146 = Bundle(w104, w217) -> (w215:cluster{dbl[], dbl[]})  [unwired: 1 in]
    n147 = Bundle(w104, w216) -> (w214:cluster{dbl[], dbl[]})  [unwired: 1 in]
    n148 = Not(x=w233) -> (.not. x?=w236:bool)
    n149 = Not(x=w230) -> (.not. x?=w231:bool)
    n150 = Select(t=w179, s="remote", f="start") -> (s? t:f=w234:bool)
    n151 = xnode "PWM"("Duty Cycle"=w240, "Frequency [Hz]"=50.0) -> ()  [unwired: 1 in, 1 out]
    n152 = xnode "PWM 2"("Duty Cycle"=w239, "Frequency [Hz]"=50.0) -> ()  [unwired: 1 in, 1 out]
    n153 = Subtract(x=360.0, y=w245) -> (x-y=w175:dbl)
    n154 = Select(t=w236, s=w234, f=w232) -> (s? t:f=w80:bool)
    n155 = Select(t=w233, s=w234, f=w232) -> (s? t:f=w81:bool)
    n156 = Select(t=w230, s=w234, f=w232) -> (s? t:f=w79:bool)
    n157 = Select(t=w231, s=w234, f=w232) -> (s? t:f=w78:bool)
    n158 = Build Array(w215, w214) -> (→"Command/Gauge":cluster{dbl[], dbl[]}[])
    n159 = Subtract(x=w175, y=0.0) -> (x-y=→"Guage":dbl)
    n160 = xnode "Digital output (1 sample)"("C/DIO6 (DIO6)"=w80, "C/DIO5 (DIO5)"=w81) -> ()  [unwired: 1 in, 1 out]
    n161 = xnode "Digital output (1 sample) 2"("C/DIO2 (DIO2)"=w79, "C/DIO1 (DIO1)"=w78) -> ()  [unwired: 1 in, 1 out]
  }
  n162 = call <vilib>:"Reset myRIO.vi"("error in (no error)"=w13) -> ()  [unwired: 10 in, 1 out]
